vi "MainV1.vi"() -> ()   [LabVIEW 2016]
uses:
  Main_Case_Control.ctl
  <vilib>/myRIO/Instrument Drivers/Onboard IO/AI/typedefs/AI Reference.ctl
  <vilib>/myRIO/Common/Instrument Driver Framework/Utilities/typedefs/myRIO Generic Hardware Reference.ctl
  <vilib>/myRIO/Common/Instrument Driver Framework/Utilities/typedefs/Hardware Version Enum.ctl
  <vilib>/myRIO/Common/Instrument Driver Framework/Utilities/typedefs/myRIO v1.0 Reference.ctl
  <vilib>/myRIO/Common/Instrument Driver Framework/Utilities/typedefs/Generic FPGA Reference.ctl
  <vilib>/myRIO/Common/Instrument Driver Framework/myRIO v1.0/AI/typedefs/AI Channels List.ctl
  <vilib>/myRIO/Common/Instrument Driver Framework/myRIO v1.0/AI/typedefs/AI Channels Enum.ctl
  <vilib>/myRIO/Common/Instrument Driver Framework/Utilities/typedefs/Analog Scaling Constants List.ctl
  <vilib>/myRIO/Common/Instrument Driver Framework/Utilities/typedefs/Analog Scaling Constants.ctl
  <vilib>/userdefined/High Color/nirio_resource_hc.ctl
  <vilib>/myRIO/Instrument Drivers/Onboard IO/PWM/typedefs/PWM Reference.ctl
  <vilib>/myRIO/Common/Instrument Driver Framework/myRIO v1.0/PWM/typedefs/PWM Channels Enum.ctl
  <vilib>/myRIO/Instrument Drivers/Onboard IO/PWM/typedefs/PWM Configuration.ctl
  <vilib>/myRIO/Common/Instrument Driver Framework/Utilities/vis/Is FPGA Ref Available.vi
  <vilib>/myRIO/Common/Instrument Driver Framework/myRIO v1.0/AI/vis/myRIO v1.1 Open AI.vi
  <vilib>/myRIO/Instrument Drivers/Onboard IO/AI/vis/Read.vi
  <vilib>/myRIO/Common/Instrument Driver Framework/myRIO v1.0/PWM/vis/myRIO v1.1 Open PWM.vi
  <vilib>/myRIO/Instrument Drivers/Onboard IO/PWM/vis/Set Duty Cycle and Frequency.vi
  <vilib>/myRIO/Common/Instrument Driver Framework/Utilities/vis/Validate Channels.vi
  <vilib>/myRIO/Common/Instrument Driver Framework/myRIO v1.0/AI/vis/myRIO v1.0 Reserve AI.vi
  <vilib>/myRIO/Common/Instrument Driver Framework/myRIO v1.0/PWM/vis/myRIO v1.0 Reserve PWM.vi
  <vilib>/myRIO/Common/Instrument Driver Framework/myRIO v1.0/AI/vis/myRIO v1.0 Build MUX Configuration AI.vi
  <vilib>/myRIO/Common/Instrument Driver Framework/myRIO v1.0/Resource Manager/vis/myRIO v1.0 Reserve Channel List.vi
  <vilib>/myRIO/Common/Instrument Driver Framework/myRIO v1.0/PWM/vis/myRIO v1.0 Build MUX Configuration PWM.vi
  <vilib>/myRIO/Common/Instrument Driver Framework/myRIO v1.0/Resource Manager/vis/myRIO v1.0 Reserve Channel.vi
  <vilib>/myRIO/Common/Instrument Driver Framework/myRIO v1.0/Resource Manager/vis/myRIO v1.0 Unreserve Channel.vi
  <vilib>/myRIO/Common/Instrument Driver Framework/myRIO v1.0/Resource Manager/vis/myRIO v1.0 Create Configuration List.vi
  <vilib>/myRIO/Common/Instrument Driver Framework/myRIO v1.0/Resource Manager/vis/myRIO v1.0 Build Mutex Name.vi
  <vilib>/Utility/VariantDataType/GetNumericInfo.vi
  <vilib>/Utility/error.llb/Error Cluster From Error Code.vi
  <vilib>/myRIO/Common/Instrument Driver Framework/myRIO v1.0/myRIO v1.1 Open.vi
  <vilib>/myRIO/Common/Instrument Driver Framework/Utilities/vis/IO Manager.vi
  <vilib>/myRIO/Common/Instrument Driver Framework/Utilities/vis/Configuration Manager.vi
  <vilib>/myRIO/Common/Instrument Driver Framework/myRIO v1.0/Resource Manager/vis/myRIO v1.0 Configure IO.vi
  <vilib>/myRIO/Common/Instrument Driver Framework/myRIO v1.0/myRIO v1.0 Close.vi
  <vilib>/myRIO/Common/Instrument Driver Framework/myRIO v1.0/PWM/vis/myRIO v1.0 Write PWM.vi
  <vilib>/myRIO/Common/Instrument Driver Framework/myRIO v1.0/AI/vis/myRIO v1.0 Get Scaling Constants AI.vi
  <vilib>/myRIO/Common/Instrument Driver Framework/myRIO v1.0/AI/vis/myRIO v1.0 Read AI.vi
  <vilib>/myRIO/Express VI/Onboard IO/PWM/PWM Express VI.xnode
  <vilib>/myRIO/Instrument Drivers/Onboard IO/PWM/vis/myRIO PWM Open.xnode
  <vilib>/myRIO/Express VI/Onboard IO/AI/AI Express VI.xnode
  <vilib>/myRIO/Instrument Drivers/Onboard IO/AI/vis/myRIO AI Open.xnode
  <vilib>/myRIO/Instrument Drivers/Onboard IO/PWM/PWM.lvlib
  <vilib>/myRIO/Instrument Drivers/Onboard IO/AI/AI.lvlib
panel:
  out "Rundenzeiten":T1
  in  "PID Lenkung IR":T2={"proportional gain (Kc)"=0.71, "integral time (Ti, min)"=2.0, "derivative time (Td, min)"=0.002} {"derivative time (Td, min)" format="%.3f"; "integral time (Ti, min)" format="%.3f"; "proportional gain (Kc)" format="%.3f"}
  out "Impulse pro Minute":dbl
  out "counter":dbl
  out "Leistung":dbl=0.07265267081512032
  out "Linefollow_Array":bool[](array[boolean])
  in  "true= folgen":bool
  in  "true = fahren":bool=TRUE
  out "Enum":T3
  in  "STOP if ON":bool
  in  "Geschwindigkeit multiplikator":dbl(knob) scale=0.0..1.0
  # "Minimum"
  # "immer nur 1 true!!!!!"
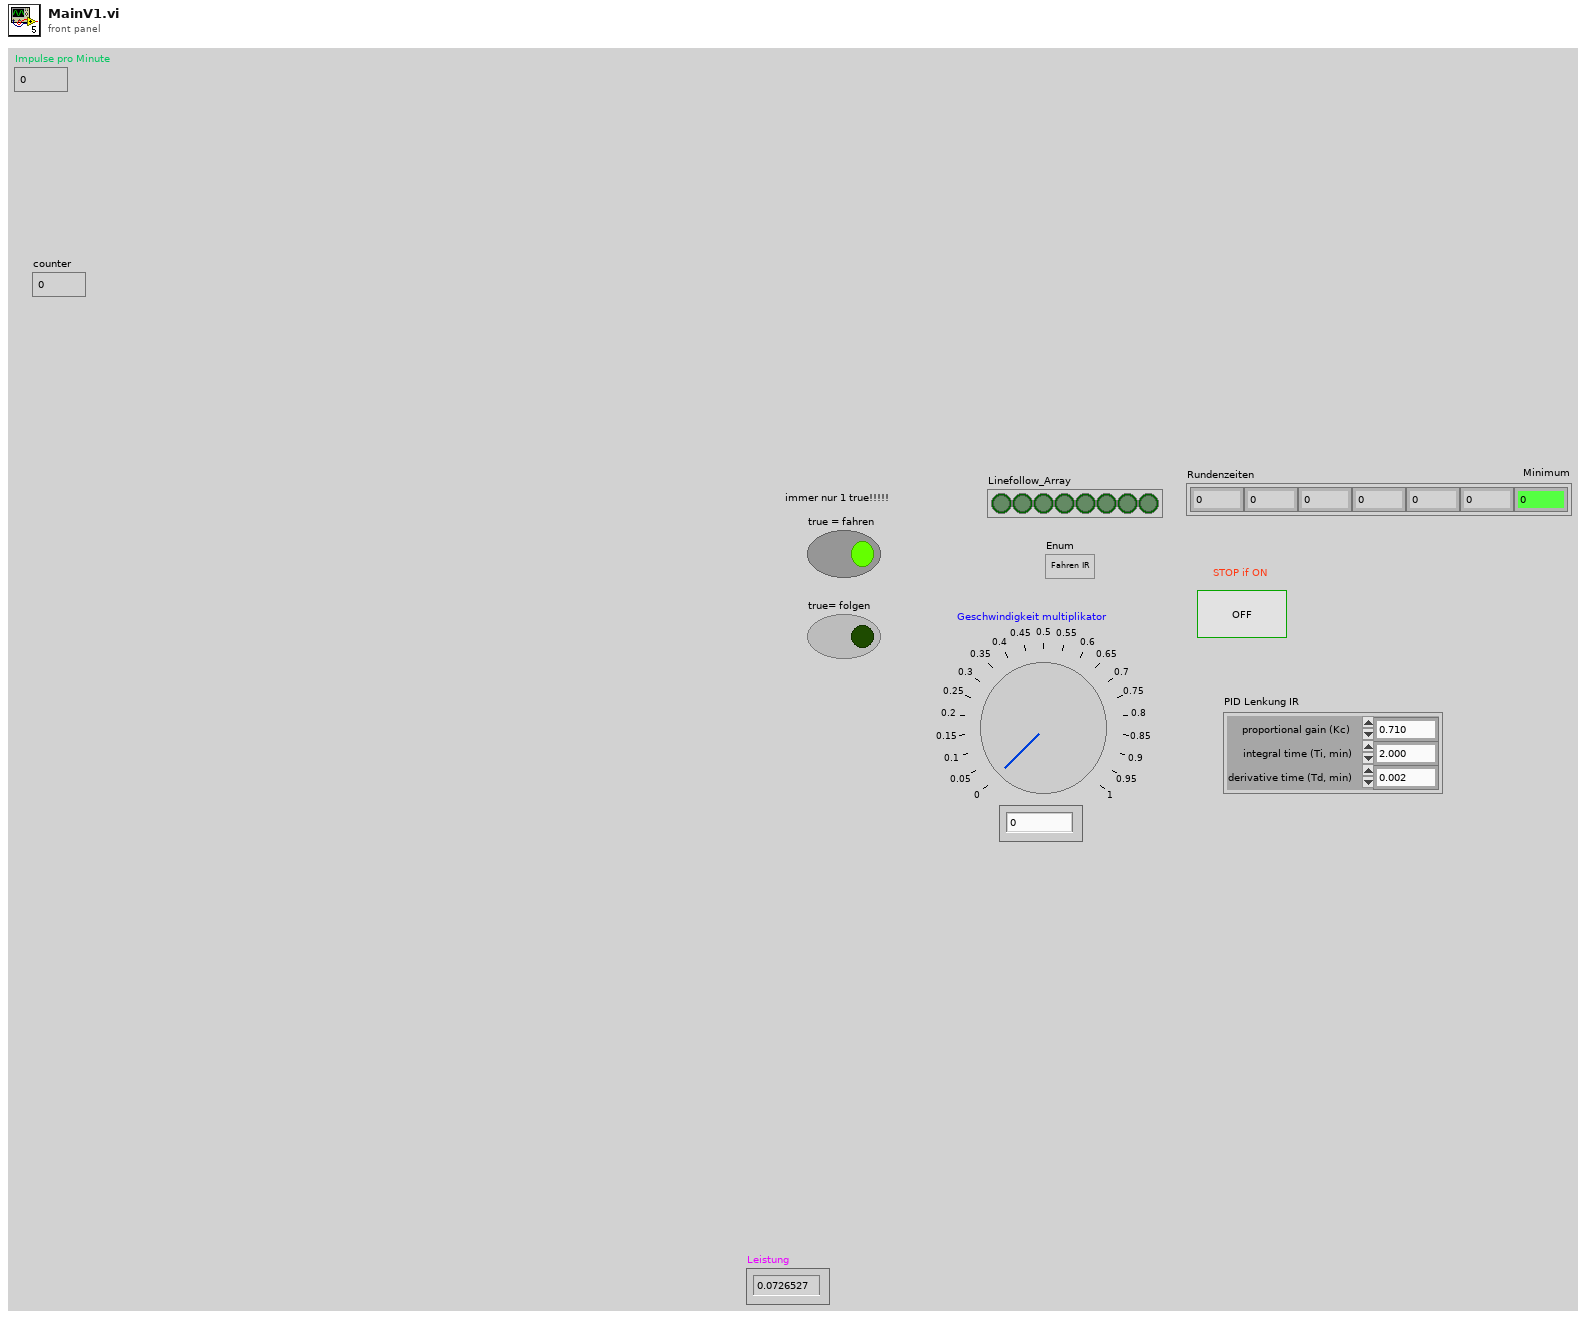
[diagram p1: front panel]
types:
  T1 = cluster{"Rundenzeiten[0]":dbl, "Rundenzeiten[1]":dbl, "Rundenzeiten[2]":dbl, "Rundenzeiten[3]":dbl, "Rundenzeiten[4]":dbl, "Rundenzeiten[5]":dbl, "Rundenzeiten[8]":dbl}
  T2 = cluster{"proportional gain (Kc)":dbl, "integral time (Ti, min)":dbl, "derivative time (Td, min)":dbl}
  T3 = typedef "Main_Case_Control.ctl" = enum16{"Fahren IR", "Fahren Array", "Folgen", "Überholen"}
  T4 = typedef "PWM.lvlib/PWM Reference.ctl" = cluster{"myRIO Reference":T5, "PWM Channels Enum":T9, "PWM Configuration":T10}
  T5 = typedef "myRIO Generic Hardware Reference.ctl" = cluster{"myRIO Model":T6, "myRIO Hardware Reference":T7}
  T6 = typedef "Hardware Version Enum.ctl" = enum16{"Unknown", "myRIO-1900", "myRIO-1950", "roboRIO", "NI ELVIS RIO CM"}
  T7 = typedef "myRIO v1.0 Reference.ctl" = cluster{"Generic FPGA Reference":T8, "Allow multiple opens":bool}
  T8 = typedef "Generic FPGA Reference.ctl" = refnum<k20>
  T9 = typedef "PWM Channels Enum.ctl" = enum16{"Not Connected", "C/PWM0", "C/PWM1", "A/PWM0", "A/PWM1", "A/PWM2", "B/PWM0", "B/PWM1", "B/PWM2", "PWM/PWM0", "PWM/PWM1", "PWM/PWM2", "PWM/PWM3", "PWM/PWM4", "PWM/PWM5", "PWM/PWM6", "PWM/PWM7", "PWM/PWM8", "PWM/PWM9"}
  T10 = typedef "PWM.lvlib/PWM Configuration.ctl" = cluster{"Frequency":dbl, "Duty Cycle":dbl}
  T11 = typedef "nirio_resource_hc.ctl" = tag
  T12 = cluster{"Rundenzeiten[0]":dbl, "Rundenzeiten[1]":dbl, "Rundenzeiten[2]":dbl, "Rundenzeiten[3]":dbl, "Rundenzeiten[4]":dbl, "Rundenzeiten[5]":dbl, "Rundenzeiten[6]":dbl}
  T13 = typedef "AI.lvlib/AI Reference.ctl" = cluster{"myRIO Reference":T5, "AI Channels List":T14, "AI Scaling Constants List":T16}
  T14 = typedef "AI Channels List.ctl" = T15[]
  T15 = typedef "AI Channels Enum.ctl" = enum16{"Not Connected", "AudioIn/Left", "AudioIn/Right", "C/AI0", "C/AI1", "A/AI0", "A/AI1", "A/AI2", "A/AI3", "B/AI0", "B/AI1", "B/AI2", "B/AI3", "AI/AI0", "AI/AI1", "AI/AI2", "AI/AI3"}
  T16 = typedef "Analog Scaling Constants List.ctl" = T17[]
  T17 = typedef "Analog Scaling Constants.ctl" = cluster{"LSB Weight (Volts)":dbl, "Offset (Volts)":dbl, "Signed?":bool}
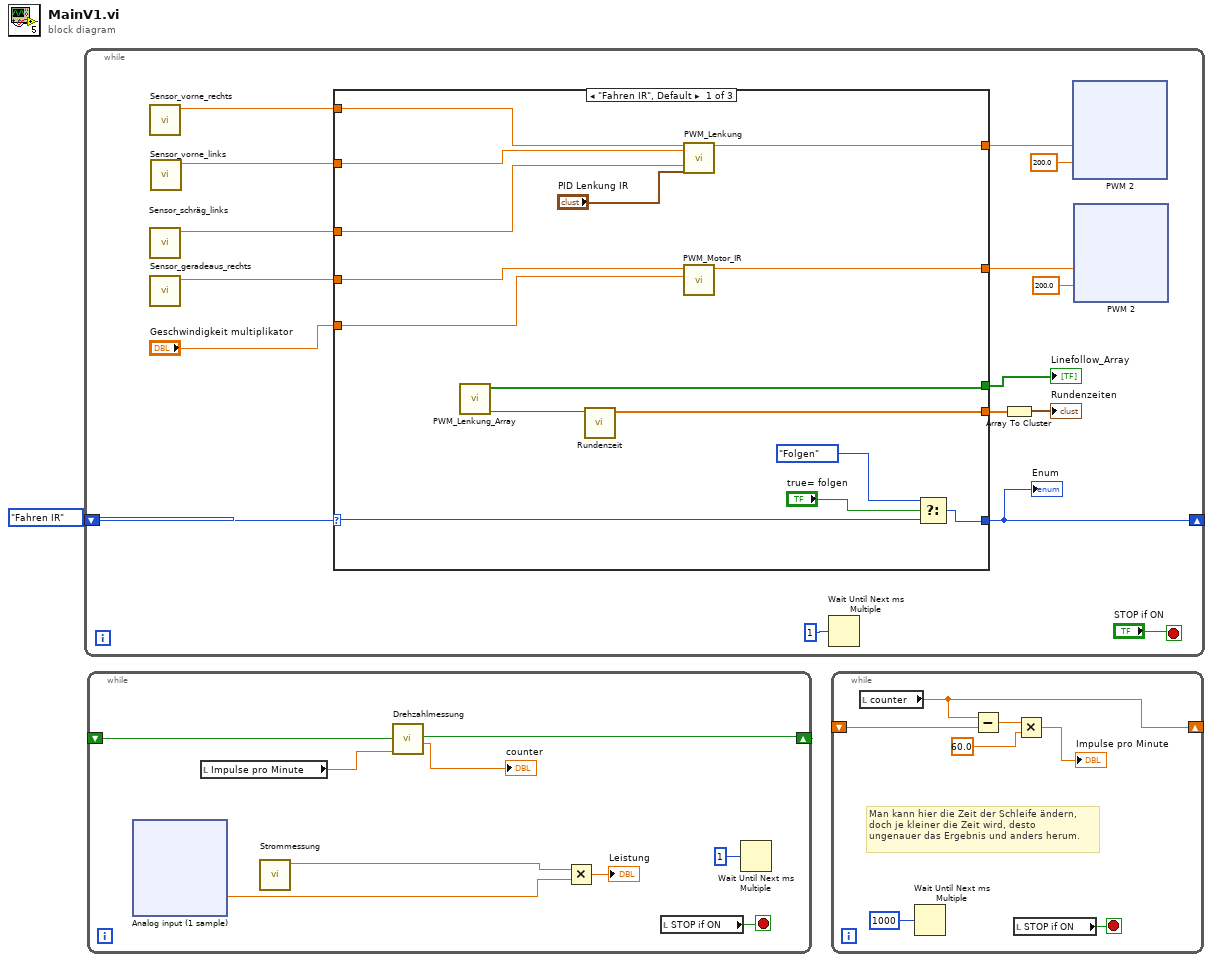
[diagram p0: block diagram]
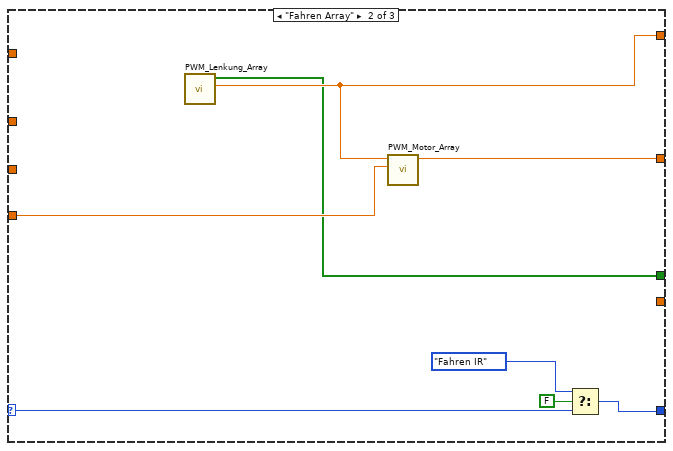
[diagram p2: hidden frame]
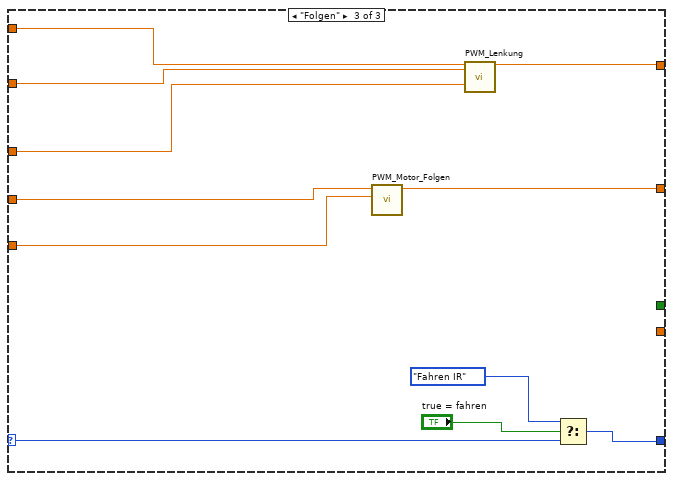
[diagram p3: hidden frame]
diagram:
  n1 = while {
    shift-right: [w13] -> _
    shift-left: Main_Case_Control."Fahren IR" -> [w14]
    stop <- "STOP if ON" stop-if-true
    n2 = call "Sensor_vorne_rechts.vi"() -> ("Abstand in cm"=w8:dbl)  [unwired: 11 in]
    n3 = call "Sensor_schräg_links.vi"() -> ("Abstand in cm"=w6:dbl)  [unwired: 11 in]
    n4 = call "Sensor_geradeaus_rechts.vi"() -> ("Abstand in cm"=w5:dbl)  [unwired: 11 in]
    n5 = call "Sensor_vorne_links.vi"() -> ("Abstand in cm"=w7:dbl)  [unwired: 11 in]
    n6 = case shown="\"Fahren IR\", Default" w14 {
      selector: w14 -> [w97 w105 w115]
      tunnel: "Geschwindigkeit multiplikator" -> [w96 w109 w116]
      tunnel: [w102 w107 w120] -> w13
      tunnel: [w100 w108 w117] -> w11
      tunnel: [w99 w110 w118] -> w9
      tunnel: w8 -> [w95 _ w114]
      tunnel: w7 -> [w94 _ w113]
      tunnel: w6 -> [w93 _ w112]
      tunnel: w5 -> [w92 _ w111]
      tunnel: [w91 _ _] -> w3
      tunnel: [w89 w103 _] -> w4
      frame "Fahren IR", Default {
        n7 = call "PWM_Lenkung_Array.vi"() -> ("8 IR true"=w88:bool, "Linefollow_Array"=w89:bool[])  [unwired: 8 in, 1 out]
        n8 = call "Rundenzeit.vi"("8 IR true"=w88) -> ("Rundenzeiten"=w91:dbl[])  [unwired: 10 in]
        n9 = call "PWM_Lenkung.vi"("vorne rechts"=w95, "vorne links"=w94, "Schräg links"=w93, "PID Lenkung"="PID Lenkung IR") -> ("PWM Lenkung"=w99:dbl)  [unwired: 15 in]
        n10 = call "PWM_Motor_IR.vi"("Sensorwert"=w92, "Geschwindigkeit multiplikator"=w96) -> ("PWM Motor"=w100:dbl)  [unwired: 6 in, 1 out]
        n11 = Select(t=Main_Case_Control."Folgen", s="true= folgen", f=w97) -> (s? t:f=w102:T3)
      }
      frame "Fahren Array" {
        n12 = call "PWM_Lenkung_Array.vi"() -> ("PWM Lenkung"=w110:dbl, "Linefollow_Array"=w103:bool[])  [unwired: 8 in, 1 out]
        n13 = call "PWM_Motor_Array.vi"("Geschwindigkeit\nmultiplikator"=w109, "PWM Sensor"=w110) -> ("PWM Motor"=w108:dbl)  [unwired: 9 in]
        n14 = Select(t=Main_Case_Control."Fahren IR", s=FALSE, f=w105) -> (s? t:f=w107:T3)
      }
      frame "Folgen" {
        n15 = call "PWM_Motor_Folgen.vi"("Geschw_IR_vorne"=w111, "Geschwindigkeit\nmultiplikator"=w116) -> ("PWM Lenkung"=w117:dbl)  [unwired: 8 in]
        n16 = call "PWM_Lenkung.vi"("vorne rechts"=w114, "vorne links"=w113, "Schräg links"=w112) -> ("PWM Lenkung"=w118:dbl)  [unwired: 16 in]
        n17 = Select(t=Main_Case_Control."Fahren IR", s="true = fahren", f=w115) -> (s? t:f=w120:T3)
      }
    }
    "Enum" <- w13
    "Linefollow_Array" <- w4
    n18 = Wait Until Next ms Multiple(millisecond multiple=u32 1) -> ()  [unwired: 1 out]
    n19 = Array To Cluster(array=w3) -> (cluster=→"Rundenzeiten":T12)
    n20 = xnode "PWM 2"("Duty Cycle"=w9, "Frequency [Hz]"=200.0 ("y")) -> ()  [unwired: 1 in, 1 out]
    n21 = xnode "PWM 2"("Duty Cycle"=w11, "Frequency [Hz]"=200.0) -> ()  [unwired: 1 in, 1 out]
  }
  n22 = while {
    shift-right: [w127] -> _
    shift-left: _ -> [w124]
    stop <- w122 stop-if-true
    n23 = xnode "Analog input (1 sample)"() -> ("C/AI0 (AI0)"=w126:dbl)  [unwired: 1 in, 1 out]
    n24 = local read "Impulse pro Minute"() -> (w129:dbl)
    n25 = call "Strommessung.vi"() -> ("Strom"=w123:dbl)  [unwired: 10 in, 1 out]
    n26 = call "Drehzahlmessung.vi"("Impuls per Minute"=w129, "in"=w124) -> ("counter"=→"counter":dbl, "out"=w127:bool)  [unwired: 6 in, 1 out]
    n27 = Multiply(x=w123, y=w126) -> (x*y=→"Leistung":dbl)
    n28 = local read "STOP if ON"() -> (w122:bool)
    n29 = Wait Until Next ms Multiple(millisecond multiple=u32 1 ("milliseconds to wait")) -> ()  [unwired: 1 out]
  }
  n30 = while {
    shift-right: [w173] -> _
    shift-left: _ -> [w172]
    stop <- w169 stop-if-true
    # "Man kann hier die Zeit der Schleife ändern, \ndoch je kleiner die Zeit wird, desto\nungenauer das Ergebnis und anders herum."
    n31 = local read "counter"() -> (w173:dbl)
    n32 = Wait Until Next ms Multiple(millisecond multiple=u32 1000 ("Vielfache von ms")) -> ()  [unwired: 1 out]
    n33 = Subtract(x=w173, y=w172) -> (x-y=w170:dbl)
    n34 = local read "STOP if ON"() -> (w169:bool)
    n35 = Multiply(x=w170, y=60.0) -> (x*y=→"Impulse pro Minute":dbl)
  }
